vi "SetTetColors.vi"(6 "Photodiode":i32, 8 "error in (no error)":errorcluster, 9 "Unsorted Tet Nums":i32[](array[numeric]), 10 "WFChart Refnum":refnum<vi>, 11 "DisplayTetrodes in":refnum<class "DisplayTetrodes.lvclass">) -> (0 "error out":errorcluster, 3 "DisplayTetrodes out":refnum<class "DisplayTetrodes.lvclass">)   [LabVIEW 2010, in "DisplayTetrodes.lvclass"]
uses:
  DisplayTetrodes.lvclass
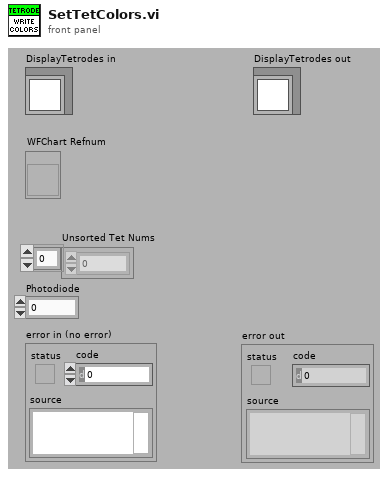
[diagram p1: front panel]
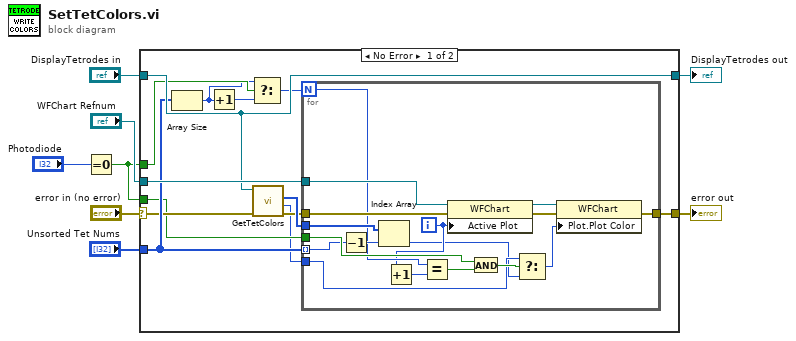
[diagram p0: block diagram]
diagram:
  n1 = Equal To 0?(x="Photodiode") -> (x = 0?=w1:bool)
  n2 = case shown="No Error" "error in (no error)" {
    selector: "error in (no error)" -> [w17 w40]
    tunnel: [w15 w40] -> w7
    tunnel: [w20 w39] -> w5
    tunnel: "DisplayTetrodes in" -> [w20 w39]
    tunnel: "WFChart Refnum" -> [w21 _]
    tunnel: "Unsorted Tet Nums" -> [w18 _]
    tunnel: w1 -> [w14 _]
    tunnel: w1 -> [w10 _]
    frame No Error {
      n3 = Array Size(array=w18) -> (size(s)=w13:i32)
      n4 = Increment(x=w13) -> (x+1=w12:i32)
      n5 = Select(t=w13, s=w14, f=w12) -> (s? t:f=w11:i32)
      n6 = call-dynamic "GetTetColors.vi"("error in (no error)"=w17, "DisplayTetrodes in"=w20) -> ("error out"=w16:errorcluster, "Photodiode"=w9:u32, "Tet Colors"=w19:u32[])  [unwired: 6 in, 1 out]
      n7 = for {
        N: w11 -> [w25]
        tunnel: w21 -> [w38]
        tunnel: w19 -> [w35]
        tunnel: w18 -> [w28] mode=indexing
        tunnel: w16 -> [w34]
        tunnel: [w32] -> w15
        tunnel: w10 -> [w30]
        tunnel: w9 -> [w23]
        i -> [w24]
        n8 = Decrement(x=w28) -> (x-1=w36:i32)
        n9 = Index Array(array=w35, index=w36) -> (element=w22:u32)
        n10 = Increment(x=w24) -> (x+1=w27:i32)
        n11 = Equal?(x=w25, y=w27) -> (x = y?=w26:bool)
        n12 = property class="WFChart"(reference=w38, error in=w34, "Active Plot"=w24) -> (reference out=w37:refnum<vi>, error out=w33:errorcluster)
        n13 = And(x=w30, y=w26) -> (x .and. y?=w29:bool)
        n14 = Select(t=w23, s=w29, f=w22) -> (s? t:f=w31:u32)
        n15 = property class="WFChart"(reference=w37, error in=w33, "Plot.Plot Color"=w31) -> (error out=w32:errorcluster)  [unwired: 1 out]
      }
    }
    frame Error {
    }
  }
  "error out" <- w7
  "DisplayTetrodes out" <- w5
